vi "Test_Results.vi"() -> ()   [LabVIEW 2025]
panel:
  out "Cluster indicator":T1
  in  "Cluster control":T2
  in  "Exit":bool caption="Save"
  in  "Save":bool
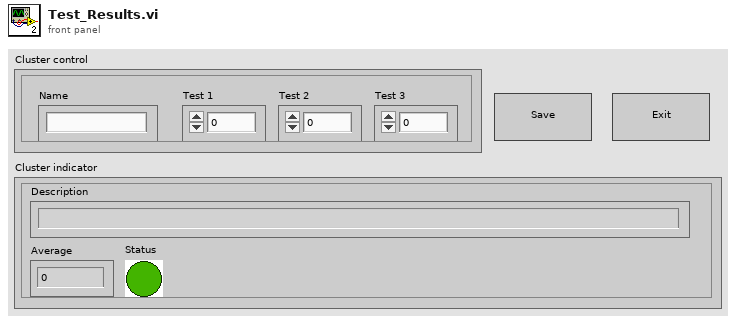
[diagram p1: front panel]
types:
  T1 = cluster{"Description":string, "Average":dbl, "Status":bool}
  T2 = cluster{"Name":string, "Test 1":dbl, "Test 2":dbl, "Test 3":dbl}
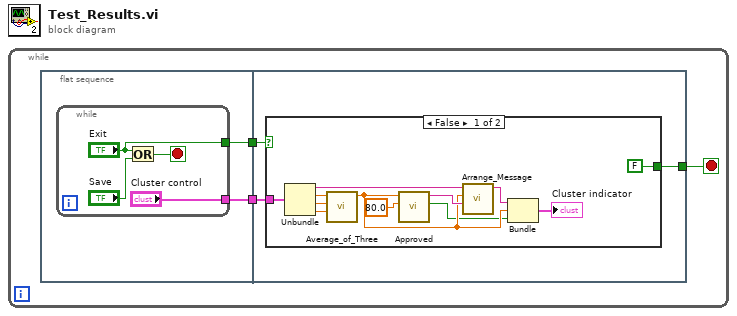
[diagram p0: block diagram]
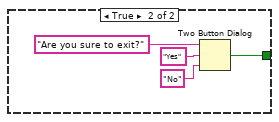
[diagram p2: hidden frame]
diagram:
  n1 = while {
    stop <- w2 stop-if-true
    n2 = flat-sequence {
      tunnel: [w5] -> w3
      tunnel: [w4] -> w1
      tunnel: w3 -> [w12]
      tunnel: [w11] -> w2
      tunnel: w1 -> [w10]
      frame #0 {
        n3 = while {
          tunnel: ["Exit"] -> w5
          tunnel: ["Cluster control"] -> w4
          stop <- w8 stop-if-true
          n4 = Or(x="Exit", y="Save") -> (x .or. y?=w8:bool)
        }
      }
      frame #1 {
        n5 = case shown="False" w12 {
          tunnel: [FALSE ("T button?") w25] -> w11
          tunnel: w10 -> [w21 _]
          frame False {
            n6 = Unbundle(w21) -> ("Name"=w20:string, "Test 1"=w19:dbl, "Test 2"=w18:dbl, "Test 3"=w17:dbl)
            n7 = call "Average_of_Three.vi"("Test 3"=w17, "Test 2"=w18, "Test 1"=w19) -> ("Average"=w15:dbl)  [unwired: 8 in]
            n8 = call "Approved.vi"("Pass value"=80.0 ("y"), "Average"=w15) -> ("Status"=w14:bool, "Approved?"=w23:string)  [unwired: 8 in]
            n9 = call "Arrange_Message.vi"("Approved?"=w23, "Average"=w15, "Name"=w20) -> ("Description"=w16:string)  [unwired: 8 in]
            n10 = Bundle("Description"=w16, "Average"=w15, "Status"=w14) -> (→"Cluster indicator":T1)  [unwired: 1 in]
          }
          frame True {
            n11 = Two Button Dialog(message="Are you sure to exit?", 1:"No" ("F button name (\"Cancel\")"), 2:"Yes" ("T button name (\"OK\")")) -> (T button?=w25:bool)
          }
        }
      }
    }
  }
